vi "DisableDissconnectButton.vi"(8 "error in (no error)":errorcluster, 10 "Disabled":T1(ring), 11 "TCP_serverGUI in":refnum<class "TCP_serverGUI.lvclass">) -> (0 "error out":errorcluster, 3 "TCP_serverGUI out":refnum<class "TCP_serverGUI.lvclass">)   [LabVIEW 2023, in "TCP_serverGUI.lvlib" / "TCP_serverGUI.lvclass"]
uses:
  TCP_serverGUI.lvclass
  TCP_serverGUI.lvclass/TCP_serverGUI.ctl
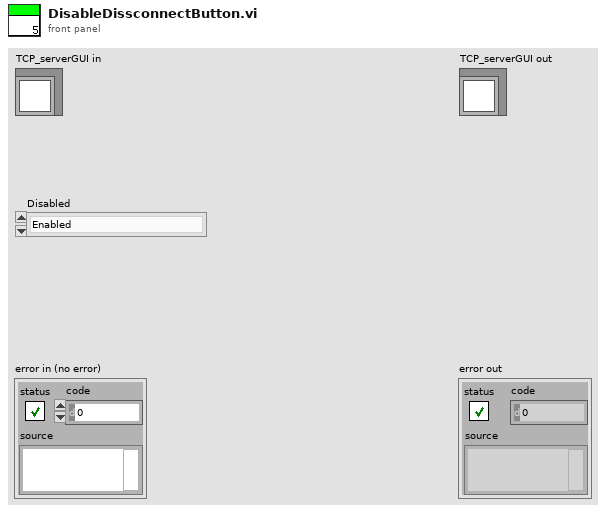
[diagram p1: front panel]
types:
  T1 = enum8{"Enabled", "Disabled", "Disabled and Grayed Out"}
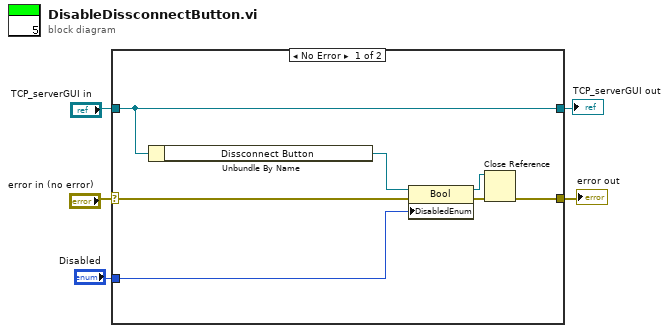
[diagram p0: block diagram]
diagram:
  n1 = case shown="No Error" "error in (no error)" {
    selector: "error in (no error)" -> [w7 w14]
    tunnel: [w6 w14] -> w4
    tunnel: [w12 w13] -> w2
    tunnel: "TCP_serverGUI in" -> [w12 w13]
    tunnel: "Disabled" -> [w10 _]
    frame No Error {
      n2 = Unbundle By Name(w12) -> ("Dissconnect Button"=w11:refnum<vi>)
      n3 = property class="Bool"(reference=w11, error in=w7, "DisabledEnum"=w10) -> (reference out=w8:refnum<vi>, error out=w9:errorcluster)
      n4 = Close Reference(reference=w8, error in (no error)=w9) -> (error out=w6:errorcluster)
    }
    frame Error {
    }
  }
  "error out" <- w4
  "TCP_serverGUI out" <- w2
